vi "Command Drive Distance.vi"(6 "Timeout":dbl=5.0, 8 "Speed":dbl=0.35, 9 "Heading":dbl=-60.0, 10 "Distance(Feet)":dbl=4.0, 11 "Startup":bool) -> (0 "Angular":dbl, 1 "Reinit":bool, 2 "Linear":dbl, 3 "Completed":bool=TRUE)   [LabVIEW 2019]
uses:
  Auto Utilities/Command_Execution_State.ctl
  Globals/Sensor_Values.vi
panel:
  in  "Turn I":dbl=0.0001
  in  "Turn D":dbl=0.005
  out "Turning":cluster{"Heading":dbl, "Drive_IMU":dbl}(graph)={"Heading"=-60.0, "Drive_IMU"=-65.830078125}
  in  "Turn P":dbl=0.03
  in  "Distance Gain":dbl=0.01
  # "Alpha .06"
  # "Beta .1"
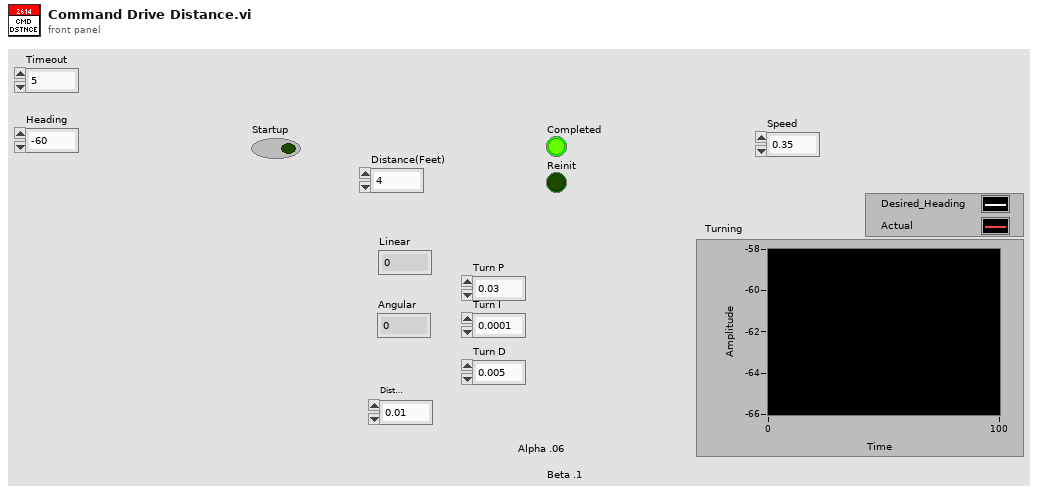
[diagram p1: front panel]
types:
  T1 = typedef "Command_Execution_State.ctl" = enum16{"Initialize", "Execute", "Finish"}
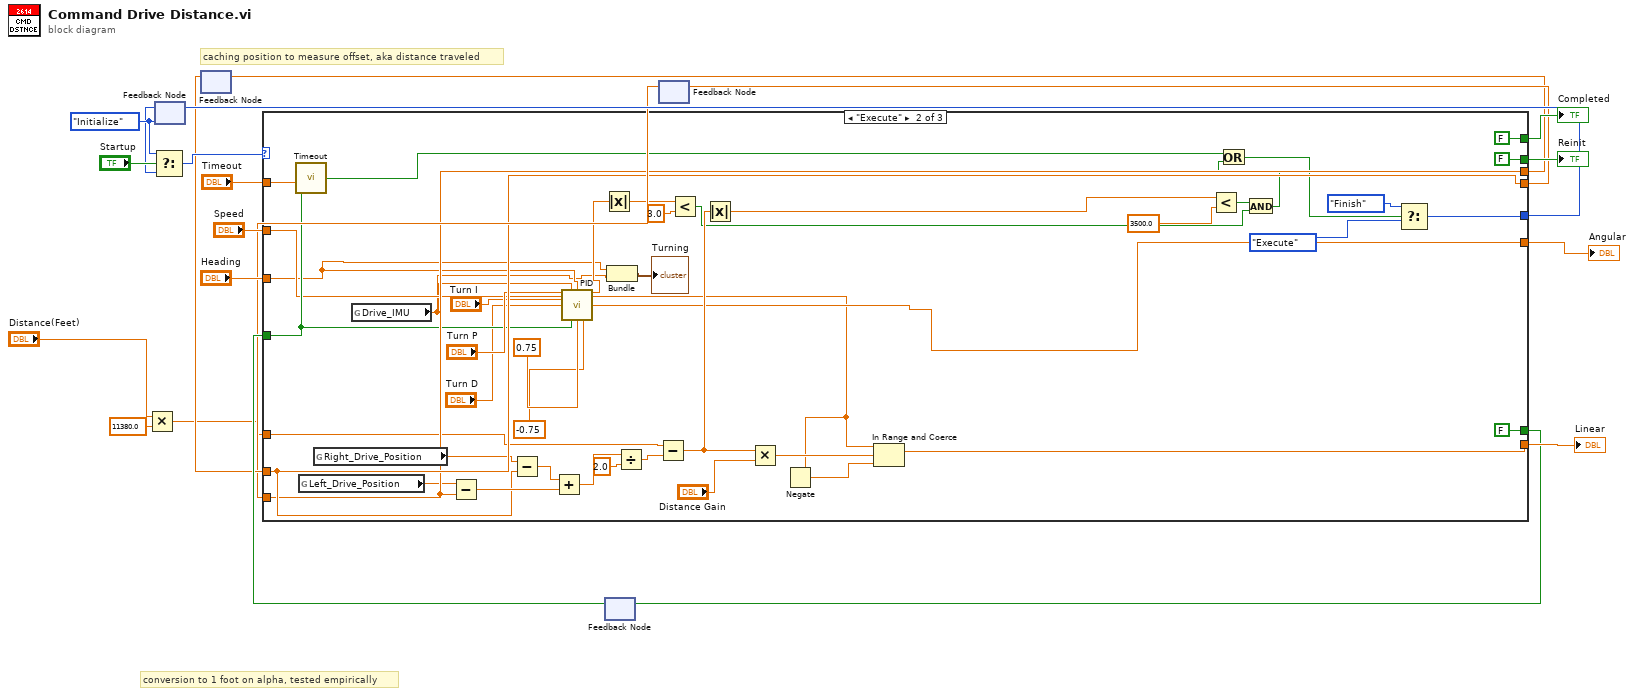
[diagram p0: block diagram]
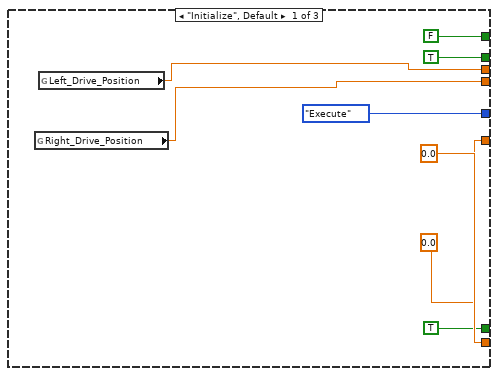
[diagram p2: hidden frame]
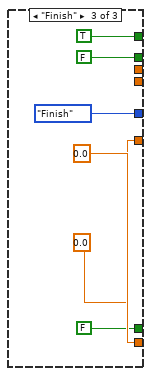
[diagram p3: hidden frame]
diagram:
  w19 = Command_Execution_State."Initialize"
  # "conversion to 1 foot on alpha, tested empirically"
  # "caching position to measure offset, aka distance traveled"
  n1 = Multiply(x="Distance(Feet)", y=11380.0) -> (x*y=w1:dbl)
  n2 = feedback #1(w19) -> (w15:T1)
  n3 = Select(t=w19, s="Startup", f=w15) -> (s? t:f=w20:T1)
  n4 = feedback #2() -> (w5:dbl)  [unwired: 1 in]
  n5 = feedback #3() -> (w10:bool)  [unwired: 1 in]
  n6 = feedback #4() -> (w4:dbl)  [unwired: 1 in]
  n7 = case shown="\"Execute\"" w20 {
    tunnel: [FALSE FALSE TRUE] -> w18
    tunnel: [TRUE FALSE FALSE] -> w17
    tunnel: [Command_Execution_State."Execute" w69 Command_Execution_State."Finish"] -> w16
    tunnel: [0.0 ("Left Wheel Velocity") w51 0.0] -> w14
    tunnel: [0.0 ("Right Wheel Velocity") w44 0.0] -> w13
    tunnel: "Heading" -> [_ w33 _]
    tunnel: [TRUE FALSE FALSE] -> w11
    tunnel: w10 -> [_ w45 _]
    tunnel: "Timeout" -> [_ w47 _]
    tunnel: "Speed" -> [_ w40 _]
    tunnel: [w22 w53 _] -> w7
    tunnel: [w23 w52 _] -> w6
    tunnel: w5 -> [_ w53 _]
    tunnel: w4 -> [_ w52 _]
    tunnel: w1 -> [_ w39 _]
    frame "Initialize", Default {
      n8 = global read "Sensor_Values.vi" "Right_Drive_Position"() -> (w22:dbl)
      n9 = global read "Sensor_Values.vi" "Left_Drive_Position"() -> (w23:dbl)
    }
    frame "Execute" {
      n10 = call "Timeout.vi"("Timeout"=w47, "Initialize"=w45) -> ("Timed Out?"=w36:bool)
      n11 = global read "Sensor_Values.vi" "Left_Drive_Position"() -> (w42:dbl)
      n12 = global read "Sensor_Values.vi" "Right_Drive_Position"() -> (w43:dbl)
      n13 = global read "Sensor_Values.vi" "Drive_IMU"() -> (w32:dbl)
      n14 = Subtract(x=w42, y=w52) -> (x-y=w54:dbl)
      n15 = Subtract(x=w43, y=w53) -> (x-y=w56:dbl)
      n16 = Add(x=w56, y=w54) -> (x+y=w57:dbl)
      n17 = call "PID.vi"("Kp"="Turn P", "Process Variable"=w32, "Goal"=w33, "Ki"="Turn I", "Kd"="Turn D", "Reinit"=w45, "Max Ouput"=0.75, "Min Output"=-0.75) -> ("Current Error"=w46:dbl, "Command"=w44:dbl)  [unwired: 5 in, 1 out]
      n18 = Absolute Value(x=w46) -> (abs(x)=w62:dbl)
      n19 = Bundle("Heading"=w33, "Drive_IMU"=w32) -> (→"Turning":cluster{"Heading":dbl, "Drive_IMU":dbl})  [unwired: 1 in]
      n20 = Divide(x=w57, y=2.0) -> (x/y=w58:dbl)
      n21 = Subtract(x=w39, y=w58) -> (x-y=w67:dbl)
      n22 = Less?(x=w62, y=3.0) -> (x < y?=w61:bool)
      n23 = Absolute Value(x=w67) -> (abs(x)=w68:dbl)
      n24 = Multiply(x=w67, y="Distance Gain") -> (x*y=w65:dbl)
      n25 = Negate(x=w40) -> (-x=w41:dbl)
      n26 = In Range and Coerce(upper limit=w40, x=w65, lower limit=w41) -> (coerced(x)=w51:dbl)  [unwired: 1 out]
      n27 = Less?(x=w68, y=3500.0) -> (x < y?=w38:bool)
      n28 = And(x=w38, y=w61) -> (x .and. y?=w35:bool)
      n29 = Or(x=w36, y=w35) -> (x .or. y?=w37:bool)
      n30 = Select(t=Command_Execution_State."Finish", s=w37, f=Command_Execution_State."Execute") -> (s? t:f=w69:T1)
    }
    frame "Finish" {
    }
  }
  "Completed" <- w18
  "Reinit" <- w17
  "Linear" <- w14
  "Angular" <- w13
  n31 = feedback-in #1(w16) -> ()
  n32 = feedback-in #2(w6) -> ()
  n33 = feedback-in #3(w11) -> ()
  n34 = feedback-in #4(w7) -> ()
